vi "Updater Setup Hosted or Stand-Alone.vi"(8 "error in (no error)":errorcluster, 11 "Spartan Install Path (empty)":path) -> (0 "error out":errorcluster, 3 "Hosted?":bool)   [LabVIEW 2011]
uses:
  <vilib>/Utility/config.llb/Write Key (Boolean).vi
  <vilib>/Utility/config.llb/NI_LVConfig.lvlib
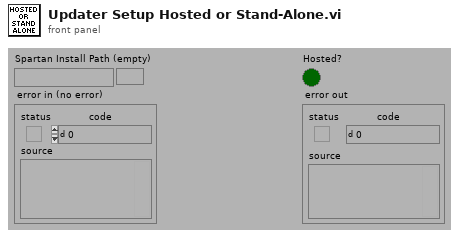
[diagram p1: front panel]
types:
  T1 = typedef "NI_LVConfig.lvlib/Config Data RefNum.ctl" = refnum<k1>
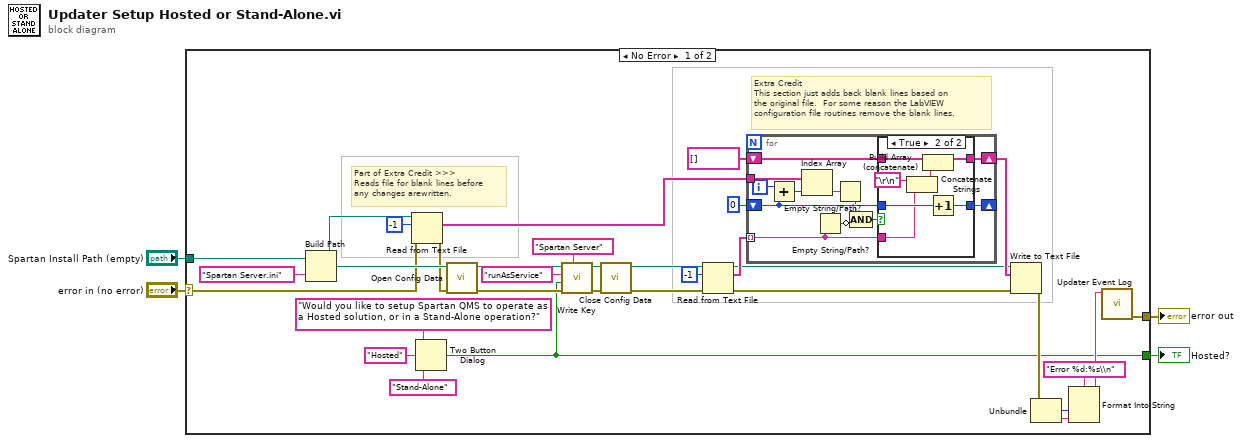
[diagram p0: block diagram]
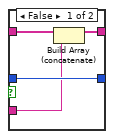
[diagram p2: hidden frame]
diagram:
  n1 = case shown="No Error" "error in (no error)" {
    selector: "error in (no error)" -> [w5 w59]
    tunnel: "Spartan Install Path (empty)" -> [w35 _]
    tunnel: [w7 w59] -> w3
    tunnel: [w6 _] -> w2
    frame No Error {
      # "Part of Extra Credit >>>\nReads file for blank lines before\nany changes arewritten."
      # "Extra Credit\nThis section just adds back blank lines based on\nthe original file.  For some reason the LabVIEW\nconfiguration file routines remove the blank lines."
      n2 = Build Path(base path=w35, name or relative path="Spartan Server.ini") -> (appended path=w17:path)
      n3 = Read from Text File(file (use dialog)=w17, count=-1, error in=w5) -> (text=w15:string[], error out=w16:errorcluster)  [unwired: 1 in, 2 out]
      n4 = Two Button Dialog(message="Would you like to setup Spartan QMS to operate as a Hosted solution, or in a Stand-Alone operation?", 1:"Stand-Alone" ("F button name (\"Cancel\")"), 2:"Hosted" ("T button name (\"OK\")")) -> (T button?=w6:bool)
      n5 = call <vilib>:"Open Config Data.vi"("error in (no error)"=w16, "configuration file path"=w17) -> ("error out"=w27:errorcluster, "refnum"=w28:T1)  [unwired: 7 in, 1 out]
      n6 = call-poly <vilib>:"Write Key.vi"("section"="Spartan Server", "error in (no error)"=w27, "value"=w6, "key"="runAsService", "refnum"=w28) -> ("error out"=w30:errorcluster, "refnum out"=w29:T1)  [unwired: 4 in, 1 out]
      n7 = call <vilib>:"Close Config Data.vi"("error in (no error)"=w30, "refnum"=w29) -> ("error out"=w13:errorcluster, "file path"=w14:path)  [unwired: 8 in]
      n8 = Read from Text File(file (use dialog)=w14, count=-1, error in=w13) -> (text=w18:string[], error out=w22:errorcluster)  [unwired: 1 in, 2 out]
      n9 = for {
        tunnel: w15 -> [w44]
        shift-right: [w46] -> w19
        shift-left: string[] [] -> [w47]
        shift-right: [w45] -> _
        shift-left: 0 -> [w41]
        tunnel: w18 -> [w38] mode=indexing
        i -> [w42]
        n10 = Add(x=w42, y=w41) -> (x+y=w40:i32)
        n11 = Index Array(array=w44, index=w40) -> (element=w43:string)
        n12 = Empty String/Path?(string/path=w38) -> (empty?=w39:bool)
        n13 = Empty String/Path?(string/path=w43) -> (empty?=w37:bool)
        n14 = Compound Arithmetic op=AND(w37, invert w39) -> (w36:bool)
        n15 = case shown="True" w36 {
          tunnel: w47 -> [w51 w58]
          tunnel: [w50 w57] -> w46
          tunnel: w41 -> [w49 w56]
          tunnel: [w49 w55] -> w45
          tunnel: w38 -> [w48 w53]
          frame False {
            n16 = Build Array (concatenate)(w51, w48) -> (w50:string[])
          }
          frame True {
            n17 = Concatenate Strings("\r\n", w53) -> (w52:string)
            n18 = Build Array (concatenate)(w58, w52) -> (w57:string[])
            n19 = Increment(x=w56) -> (x+1=w55:i32)
          }
        }
      }
      n20 = Write to Text File(file (use dialog)=w14, text=w19, error in=w22) -> (error out=w12:errorcluster)  [unwired: 1 in, 2 out]
      n21 = Unbundle(w12) -> ("code"=w10:i32, "source"=w9:string)  [unwired: 1 out]
      n22 = Format Into String(format string="Error %d:%s\\n" ("pattern"), w10, w9) -> (resulting string=w8:string)  [unwired: 2 in, 1 out]
      n23 = call "Updater Event Log.vi"("Log Entry"=w8) -> ("error out"=w7:errorcluster)  [unwired: 1 in, 9 out]
    }
    frame Error {
    }
  }
  "error out" <- w3
  "Hosted?" <- w2
